vi "valuePathv2.vi"(8 "error in (no error)":errorcluster, 10 "Array":string[](array[string]), 11 "ConsoleViewer in":refnum<class "ConsoleViewer.lvclass">) -> (0 "error out":errorcluster, 2 "Array 2":string[][](array[string]), 3 "ConsoleViewer out":refnum<class "ConsoleViewer.lvclass">)   [LabVIEW 2009, in "Views.lvlib" / "ConsoleViewer.lvclass"]
uses:
  ConsoleViewer.lvclass
  ConsoleViewer.lvclass/ConsoleViewer.ctl
  Tools/CommandProcessor/CommandEvents/CommandEvents.lvclass
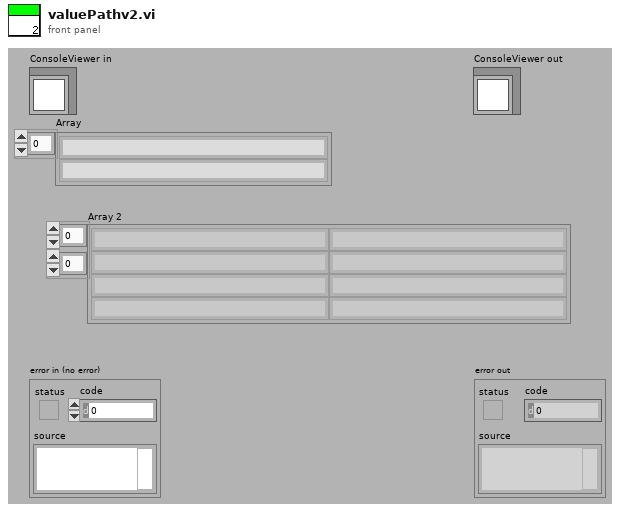
[diagram p1: front panel]
types:
  T1 = cluster{"newCommand":refnum<user-event>, "textUpdate":refnum<user-event>}
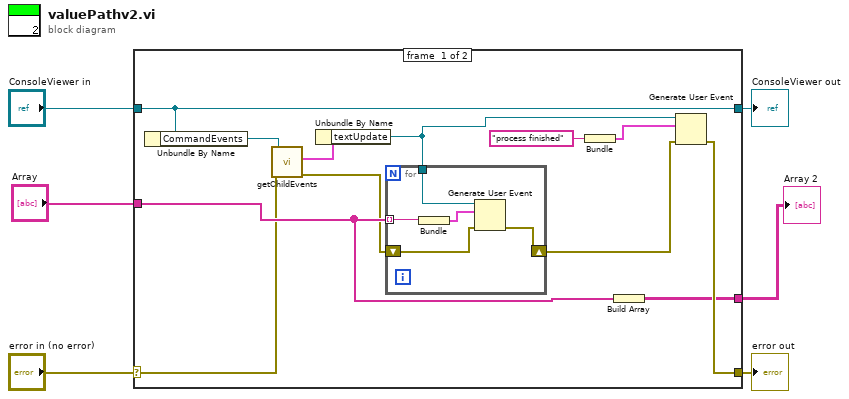
[diagram p0: block diagram]
diagram:
  n1 = case shown="No Error" "error in (no error)" {
    selector: "error in (no error)" -> [w8 w25]
    tunnel: [w11 w25] -> w5
    tunnel: [w18 w24] -> w3
    tunnel: "ConsoleViewer in" -> [w18 w24]
    tunnel: "Array" -> [w10 _]
    tunnel: [w9 _] -> w1
    frame #0 {
      n2 = Unbundle By Name(w18) -> ("CommandEvents"=w17:refnum<class "CommandEvents.lvclass">)
      n3 = call-dynamic "getChildEvents.vi"("error in (no error)"=w8, "CommandEvents in"=w17) -> ("error out"=w7:errorcluster, "Events"=w16:T1)  [unwired: 7 in, 1 out]
      n4 = Unbundle By Name(w16) -> ("textUpdate"=w13:refnum<user-event>)
      n5 = for {
        tunnel: w10 -> [w20] mode=indexing
        tunnel: w13 -> [w22]
        shift-right: [w21] -> w12
        shift-left: w7 -> [w23]
        n6 = Bundle("node"=w20) -> (w19:cluster{"node":string})  [unwired: 1 in]
        n7 = Generate User Event(user event=w22, event data cluster=w19, error in=w23) -> (error out=w21:errorcluster)  [unwired: 1 out]
      }
      n8 = Bundle("process finished") -> (w15:cluster{string})  [unwired: 1 in]
      n9 = Build Array(w10) -> (w9:string[][])
      n10 = Generate User Event(user event=w13, event data cluster=w15, error in=w12) -> (error out=w11:errorcluster)  [unwired: 1 out]
    }
    frame #1 {
    }
  }
  "error out" <- w5
  "ConsoleViewer out" <- w3
  "Array 2" <- w1
